vi "LVPortGetEventStream.vi"(8 "error in":errorcluster, 10 "Category":string, 11 "ID":string) -> (0 "error out":errorcluster, 1 "Event Stream Info":T1, 2 "Stream":refnum<user-event>, 3 "Event Registration Refnum out":refnum<event-registration>)   [LabVIEW 2017]
uses:
  LVPortEventStreamType.ctl
  LVPortEventType.ctl
  LVPortEventGlobals.vi
panel:
  out "Stream Name":string
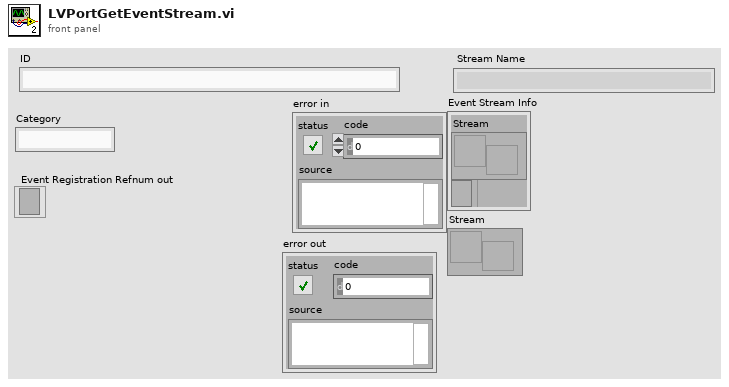
[diagram p1: front panel]
types:
  T1 = typedef "LVPortEventStreamType.ctl" = cluster{"Stream":refnum<user-event>, "Event Registration":refnum<event-registration>}
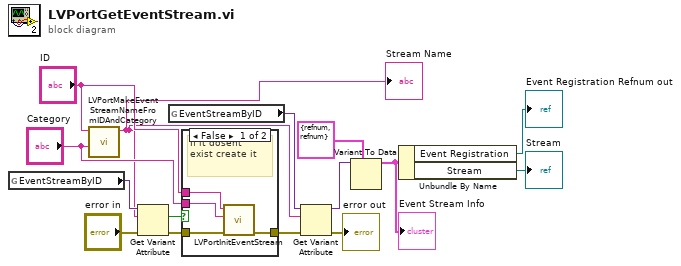
[diagram p0: block diagram]
diagram:
  n1 = global read "LVPortEventGlobals.vi" "EventStreamByID"() -> (w11:variant)
  n2 = call "LVPortMakeEventStreamNameFromIDAndCategory.vi"("Category"="Category", "ID"="ID") -> ("StreamName"=w1:string)  [unwired: 9 in]
  "Stream Name" <- w1
  n3 = Get Variant Attribute(Variant=w11, name=w1, error in="error in") -> (found=w2:bool, error out=w14:errorcluster)  [unwired: 1 in, 2 out]
  n4 = global read "LVPortEventGlobals.vi" "EventStreamByID"() -> (w10:variant)
  n5 = case shown="False" w2 {
    tunnel: w14 -> [w17 w20]
    tunnel: [w16 w20] -> w13
    tunnel: "ID" -> [w19 _]
    tunnel: "Category" -> [w18 _]
    frame False {
      # "If it dosent\nexist create it"
      n6 = call "LVPortInitEventStream.vi"("error in"=w17, "Category"=w18, "ID"=w19) -> ("error out"=w16:errorcluster)  [unwired: 7 in, 1 out]
    }
    frame True {
    }
  }
  n7 = Get Variant Attribute(Variant=w10, name=w1, error in=w13) -> (duplicate Variant=w8:variant, error out=→"error out":errorcluster)  [unwired: 1 in, 2 out]
  n8 = Variant To Data(type=T1 {"Stream"=refnum, "Event Registration"=refnum} ("EventStreamInfo"), Variant=w8) -> (data=w7:T1)  [unwired: 1 in, 1 out]
  "Event Stream Info" <- w7
  n9 = Unbundle By Name(w7) -> ("Event Registration"=→"Event Registration Refnum out":refnum<event-registration>, "Stream"=→"Stream":refnum<user-event>)
